vi "AIT 664 - Extract Input VLs from System Explorer.vi"(0 "Item Ref":T8=18446744073709551615 format="%.0x", 5 "664 End System":T1, 11 "error in (no error)":errorcluster) -> (6 "Input VLs Out":T6[](array[typedef]), 15 "error out":errorcluster)   [LabVIEW 2013, in "AIT 664 Custom Device.lvlib"]
doc: "Extract the Input VLs from the system explorer and return the parameters defined by the user"
uses:
  AIT 664 Custom Device.lvlib
  Controls/664 - XML Input VL.ctl
  Controls/664 - XML Rx Message Port.ctl
  Controls/664 - Sampling Type.ctl
  Controls/664 -Param.ctl
  <vilib>/NI Veristand/Custom Device API/Custom Device Item Ref.ctl
  Controls/664 - XML End System Description.ctl
  Controls/664 - XML Output VL.ctl
  Controls/664 - XML Tx Message Port.ctl
  Controls and Global/Global.vi
  <vilib>/NI Veristand/Custom Device Tools/Custom Device Utility Library/NI VeriStand - Search for All Items by GUID.vi
  <vilib>/NI Veristand/Custom Device API/Get Item Property (U32).vi
  <vilib>/NI Veristand/Custom Device API/Custom Device API.lvlib
  <vilib>/NI Veristand/Custom Device Tools/Custom Device Utility Library/Custom Device Utility Library.lvlib
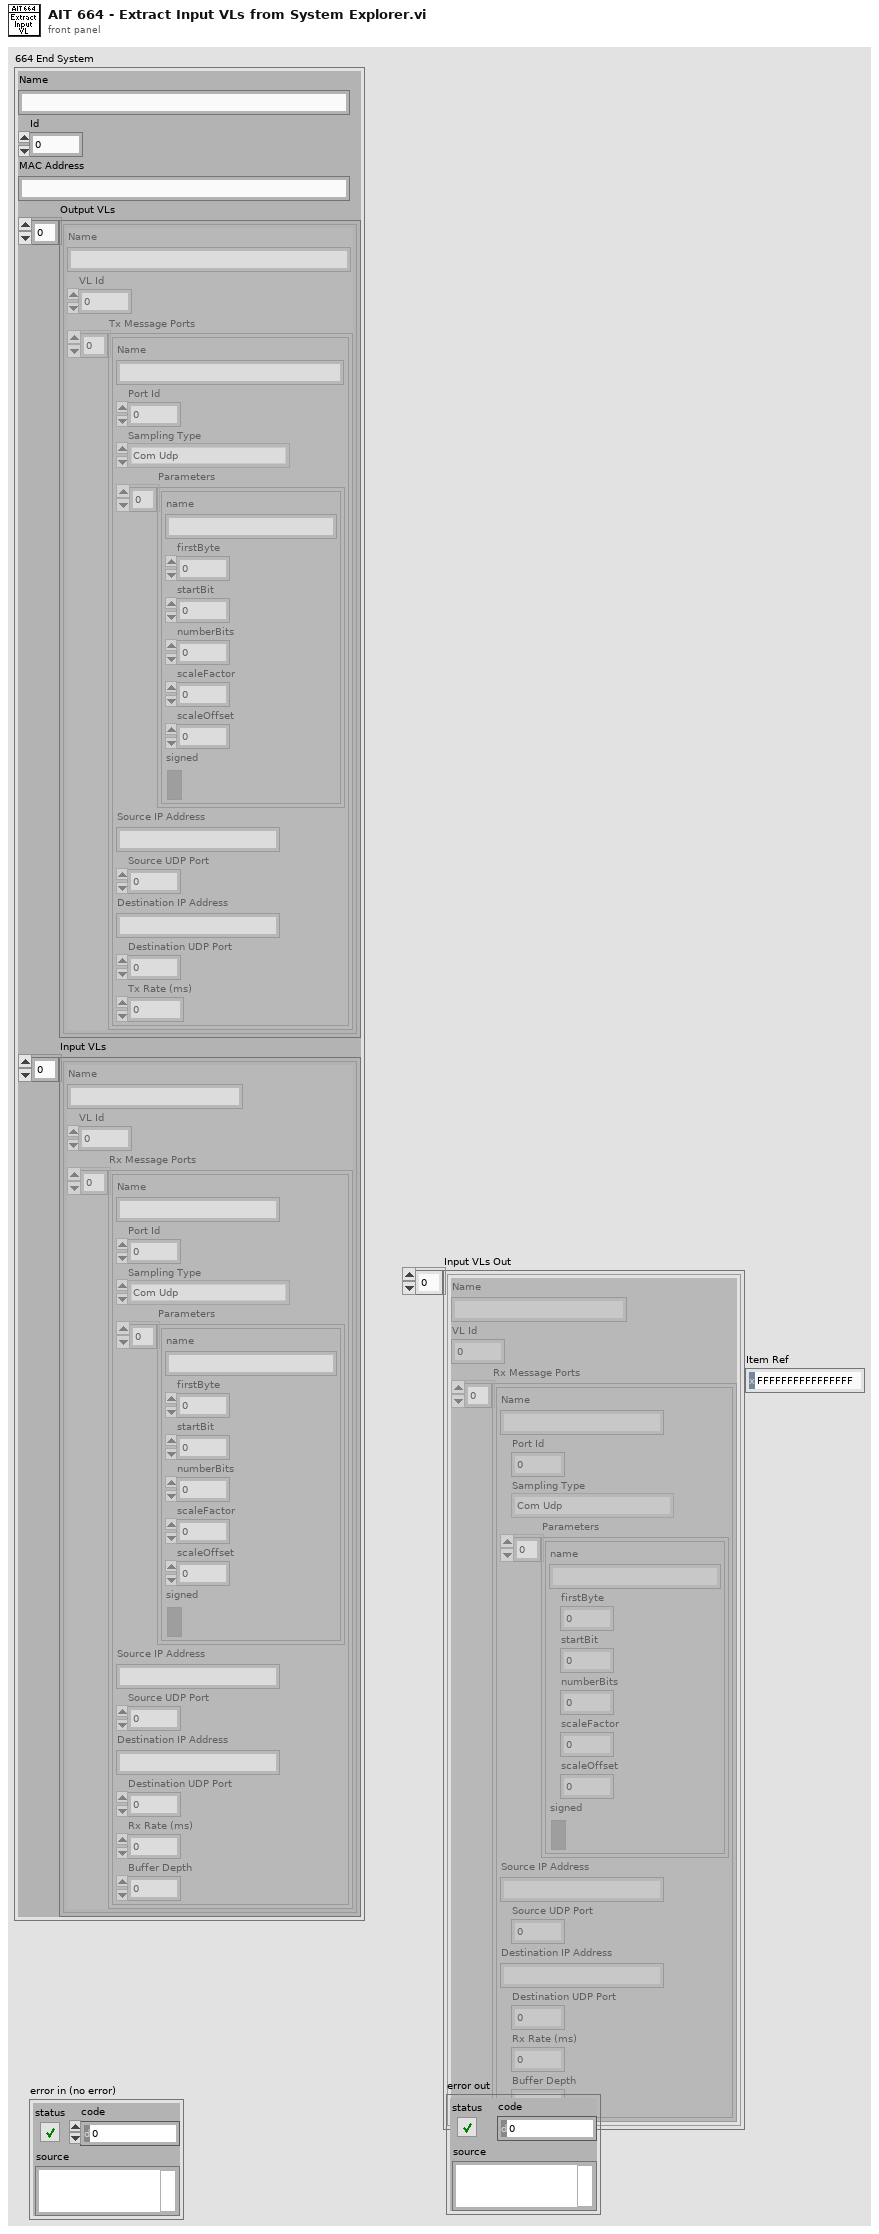
[diagram p1: front panel]
types:
  T1 = typedef "AIT 664 Custom Device.lvlib/664 - XML End System Description.ctl" = cluster{"Name":string, "Id":u32, "MAC Address":string, "Output VLs":T2[], "Input VLs":T6[]}
  T2 = typedef "AIT 664 Custom Device.lvlib/664 - XML Output VL.ctl" = cluster{"Name":string, "VL Id":u32, "Tx Message Ports":T3[]}
  T3 = typedef "AIT 664 Custom Device.lvlib/664 - XML Tx Message Port.ctl" = cluster{"Name":string, "Port Id":u32, "Sampling Type":T4, "Parameters":T5[], "Source IP Address":string, "Source UDP Port":u32, "Destination IP Address":string, "Destination UDP Port":u32, "Tx Rate (ms)":u32}
  T4 = typedef "AIT 664 Custom Device.lvlib/664 - Sampling Type.ctl" = enum16{"Com Udp", "Com Udp Queuing", "Sap Udp", "Sap Ip", "Sap Mac", "Unknown"}
  T5 = typedef "AIT 664 Custom Device.lvlib/664 -Param.ctl" = cluster{"name":string, "firstByte":i32, "startBit":i32, "numberBits":i32, "scaleFactor":dbl, "scaleOffset":dbl, "signed":bool}
  T6 = typedef "AIT 664 Custom Device.lvlib/664 - XML Input VL.ctl" = cluster{"Name":string, "VL Id":u32, "Rx Message Ports":T7[]}
  T7 = typedef "AIT 664 Custom Device.lvlib/664 - XML Rx Message Port.ctl" = cluster{"Name":string, "Port Id":u32, "Sampling Type":T4, "Parameters":T5[], "Source IP Address":string, "Source UDP Port":u32, "Destination IP Address":string, "Destination UDP Port":u32, "Rx Rate (ms)":u32, "Buffer Depth":u32}
  T8 = typedef "Custom Device API.lvlib/Custom Device Item Ref.ctl" = u64
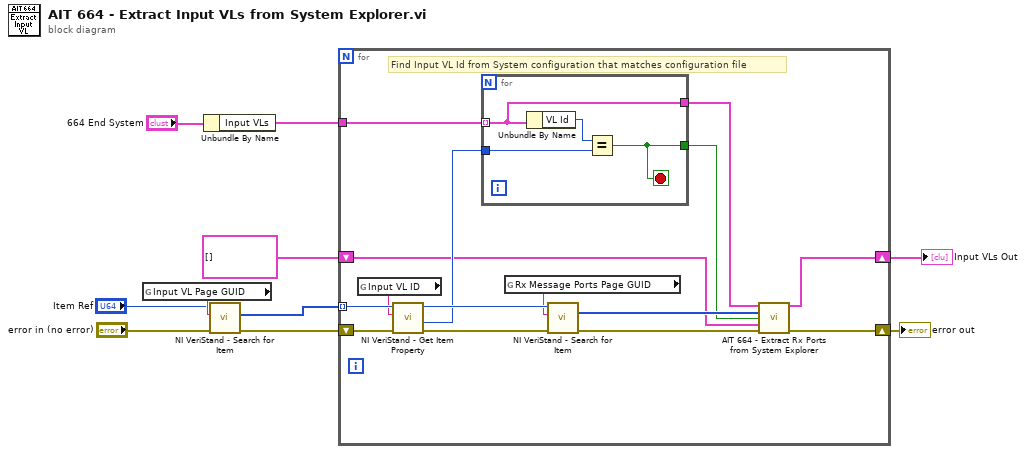
[diagram p0: block diagram]
diagram:
  n1 = global read "Global.vi" "Input VL Page GUID"() -> (w8:string)
  n2 = Unbundle By Name("664 End System") -> ("Input VLs"=w1:T6[])
  n3 = call-poly <vilib>:"NI VeriStand - Search for Item.vi"("error in"="error in (no error)", "Item GUID"=w8, "Section Ref in"="Item Ref") -> ("error out"=w6:errorcluster, "Item Refs"=w4:T8[])  [unwired: 5 in, 2 out]
  n4 = for {
    tunnel: w4 -> [w25] mode=indexing
    tunnel: w1 -> [w19]
    shift-right: [w14] -> w10
    shift-left: T6[] [] -> [w15]
    shift-right: [w12] -> w3
    shift-left: w6 -> [w11]
    # "Find Input VL Id from System configuration that matches configuration file"
    n5 = global read "Global.vi" "Input VL ID"() -> (w24:string)
    n6 = call-poly <vilib>:"NI VeriStand - Get Item Property.vi"("error in (no error)"=w11, "Property Name"=w24, "Item Ref in"=w25) -> ("error out"=w23:errorcluster, "Value"=w18:u32, "Item Ref out"=w22:T8)  [unwired: 5 in, 1 out]
    n7 = for {
      tunnel: w19 -> [w26] mode=indexing
      tunnel: w18 -> [w28]
      tunnel: [w27] -> w17
      tunnel: [w26] -> w16
      stop <- w27 stop-if-true
      n8 = Unbundle By Name(w26) -> ("VL Id"=w29:u32)
      n9 = Equal?(x=w29, y=w28) -> (x = y?=w27:bool)
    }
    n10 = global read "Global.vi" "Rx Message Ports Page GUID"() -> (w21:string)
    n11 = call-poly <vilib>:"NI VeriStand - Search for Item.vi"("error in"=w23, "Item GUID"=w21, "Section Ref in"=w22) -> ("error out"=w13:errorcluster, "Item Refs"=w20:T8[])  [unwired: 5 in, 2 out]
    n12 = call "AIT 664 - Extract Rx Ports from System Explorer.vi"("Found Input VL"=w16, "Item Refs"=w20, "VL Id Found?"=w17, "Input VLs"=w15, "error in (no error)"=w13) -> ("Input VLs in"=w14:T6[], "error out"=w12:errorcluster)  [unwired: 9 in]
  }
  "Input VLs Out" <- w10
  "error out" <- w3
